vi "EVT HLP Set Frame Param.vi"(5 "convertBitDepth":i32, 6 "convertColor":i32, 7 "pixel_type":u32, 9 "size_y":u32, 10 "size_x":u32, 11 "frame":T1) -> (3 "frame out":T1)   [LabVIEW 2019, in "EmergentCameraC.lvlib"]
doc: "EMERGENTCAMERAC_API void EVT_HLP_SetFrameParam(EmergentFrame* frame, unsigned int size_x, unsigned int size_y, PIXEL_FORMAT pixel_type, int convertColor, int convertBitDepth);"
uses:
  EmergentCameraC.lvlib
  emergentInstall_Windows/win64/eSDK/bin/EmergentCameraC.dll
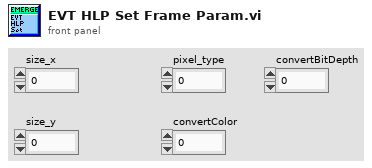
[diagram p1: front panel]
types:
  T1 = cluster{"pixel_type":u32, "size_x":u32, "size_y":u32, "stride":i32, "offset_x":u32, "offset_y":u32, "padding_x":u32, "padding_y":u32, "trailer_size_y":u32, "frame_id":u16, "@dummy control@":i8, "@dummy control@":i8, "imagePtr":i64, "bufferSize":u32, "@dummy control@":i8, "@dummy control@":i8, "@dummy control@":i8, "@dummy control@":i8, "timestamp":u64, "nsecs":u64, "convertColor":i32, "convertBitDepth":i32, "privateData[0]":u8, "privateData[1]":u8, "privateData[2]":u8, "privateData[3]":u8, "privateData[4]":u8, "privateData[5]":u8, "privateData[6]":u8, "privateData[7]":u8, "privateData[8]":u8, "privateData[9]":u8, "privateData[10]":u8, "privateData[11]":u8, "privateData[12]":u8, "privateData[13]":u8, "privateData[14]":u8, "privateData[15]":u8, "privateData[16]":u8, "privateData[17]":u8, "privateData[18]":u8, "privateData[19]":u8, "privateData[20]":u8, "privateData[21]":u8, "privateData[22]":u8, "privateData[23]":u8, "privateData[24]":u8, "privateData[25]":u8, "privateData[26]":u8, "privateData[27]":u8, "privateData[28]":u8, "privateData[29]":u8, "privateData[30]":u8, "privateData[31]":u8, "privateData[32]":u8, "privateData[33]":u8, "privateData[34]":u8, "privateData[35]":u8, "privateData[36]":u8, "privateData[37]":u8, "privateData[38]":u8, "privateData[39]":u8, "privateData[40]":u8, "privateData[41]":u8, "privateData[42]":u8, "privateData[43]":u8, "privateData[44]":u8, "privateData[45]":u8, "privateData[46]":u8, "privateData[47]":u8, "privateData[48]":u8, "privateData[49]":u8, "privateData[50]":u8, "privateData[51]":u8, "privateData[52]":u8, "privateData[53]":u8, "privateData[54]":u8, "privateData[55]":u8, "privateData[56]":u8, "privateData[57]":u8, "privateData[58]":u8, "privateData[59]":u8, "privateData[60]":u8, "privateData[61]":u8, "privateData[62]":u8, "privateData[63]":u8, "privateData[64]":u8, "privateData[65]":u8, "privateData[66]":u8, "privateData[67]":u8, "privateData[68]":u8, "privateData[69]":u8, "privateData[70]":u8, "privateData[71]":u8, "privateData[72]":u8, "privateData[73]":u8, "privateData[74]":u8, "privateData[75]":u8, "privateData[76]":u8, "privateData[77]":u8, "privateData[78]":u8, "privateData[79]":u8, "privateData[80]":u8, "privateData[81]":u8, "privateData[82]":u8, "privateData[83]":u8, "privateData[84]":u8, "privateData[85]":u8, "privateData[86]":u8, "privateData[87]":u8, "privateData[88]":u8, "privateData[89]":u8, "privateData[90]":u8, "privateData[91]":u8, "privateData[92]":u8, "privateData[93]":u8, "privateData[94]":u8, "privateData[95]":u8, "privateData[96]":u8, "privateData[97]":u8, "privateData[98]":u8, "privateData[99]":u8, "privateData[100]":u8, "privateData[101]":u8, "privateData[102]":u8, "privateData[103]":u8, "privateData[104]":u8, "privateData[105]":u8, "privateData[106]":u8, "privateData[107]":u8, "privateData[108]":u8, "privateData[109]":u8, "privateData[110]":u8, "privateData[111]":u8, "privateData[112]":u8, "privateData[113]":u8, "privateData[114]":u8, "privateData[115]":u8, "privateData[116]":u8, "privateData[117]":u8, "privateData[118]":u8, "privateData[119]":u8, "privateData[120]":u8, "privateData[121]":u8, "privateData[122]":u8, "privateData[123]":u8, "privateData[124]":u8, "privateData[125]":u8, "privateData[126]":u8, "privateData[127]":u8, "privateData[128]":u8, "privateData[129]":u8, "privateData[130]":u8, "privateData[131]":u8, "privateData[132]":u8, "privateData[133]":u8, "privateData[134]":u8, "privateData[135]":u8, "privateData[136]":u8, "privateData[137]":u8, "privateData[138]":u8, "privateData[139]":u8, "privateData[140]":u8, "privateData[141]":u8, "privateData[142]":u8, "privateData[143]":u8, "privateData[144]":u8, "privateData[145]":u8, "privateData[146]":u8, "privateData[147]":u8, "privateData[148]":u8, "privateData[149]":u8, "privateData[150]":u8, "privateData[151]":u8, "privateData[152]":u8, "privateData[153]":u8, "privateData[154]":u8, "privateData[155]":u8, "privateData[156]":u8, "privateData[157]":u8, "privateData[158]":u8, "privateData[159]":u8, "privateData[160]":u8, "privateData[161]":u8, "privateData[162]":u8, "privateData[163]":u8, "privateData[164]":u8, "privateData[165]":u8, "privateData[166]":u8, "privateData[167]":u8, "privateData[168]":u8, "privateData[169]":u8, "privateData[170]":u8, "privateData[171]":u8, "privateData[172]":u8, "privateData[173]":u8, "privateData[174]":u8, "privateData[175]":u8, "privateData[176]":u8, "privateData[177]":u8, "privateData[178]":u8, "privateData[179]":u8, "privateData[180]":u8, "privateData[181]":u8, "privateData[182]":u8, "privateData[183]":u8, "privateData[184]":u8, "privateData[185]":u8, "privateData[186]":u8, "privateData[187]":u8, "privateData[188]":u8, "privateData[189]":u8, "privateData[190]":u8, "privateData[191]":u8, "privateData[192]":u8, "privateData[193]":u8, "privateData[194]":u8, "privateData[195]":u8, "privateData[196]":u8, "privateData[197]":u8, "privateData[198]":u8, "privateData[199]":u8, "privateData[200]":u8, "privateData[201]":u8, "privateData[202]":u8, "privateData[203]":u8, "privateData[204]":u8, "privateData[205]":u8, "privateData[206]":u8, "privateData[207]":u8, "privateData[208]":u8, "privateData[209]":u8, "privateData[210]":u8, "privateData[211]":u8, "privateData[212]":u8, "privateData[213]":u8, "privateData[214]":u8, "privateData[215]":u8, "privateData[216]":u8, "privateData[217]":u8, "privateData[218]":u8, "privateData[219]":u8, "privateData[220]":u8, "privateData[221]":u8, "privateData[222]":u8, "privateData[223]":u8, "privateData[224]":u8, "privateData[225]":u8, "privateData[226]":u8, "privateData[227]":u8, "privateData[228]":u8, "privateData[229]":u8, "privateData[230]":u8, "privateData[231]":u8, "privateData[232]":u8, "privateData[233]":u8, "privateData[234]":u8, "privateData[235]":u8, "privateData[236]":u8, "privateData[237]":u8, "privateData[238]":u8, "privateData[239]":u8, "privateData[240]":u8, "privateData[241]":u8, "privateData[242]":u8, "privateData[243]":u8, "privateData[244]":u8, "privateData[245]":u8, "privateData[246]":u8, "privateData[247]":u8, "privateData[248]":u8, "privateData[249]":u8, "privateData[250]":u8, "privateData[251]":u8, "privateData[252]":u8, "privateData[253]":u8, "privateData[254]":u8, "privateData[255]":u8}
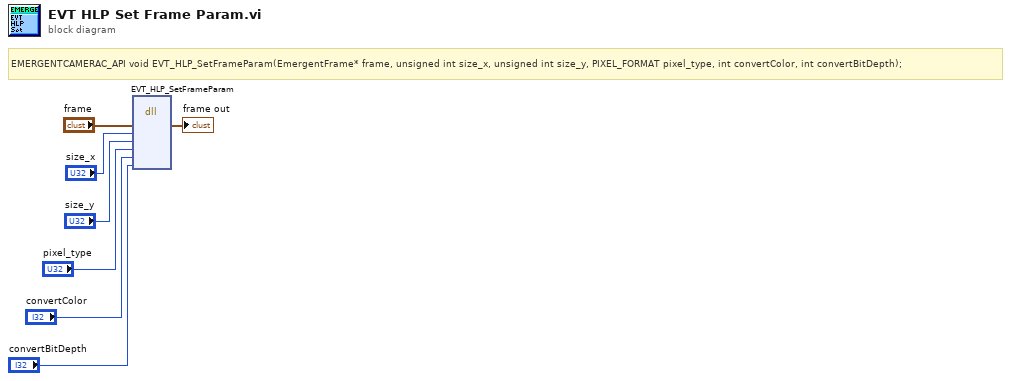
[diagram p0: block diagram]
diagram:
  # "EMERGENTCAMERAC_API void EVT_HLP_SetFrameParam(EmergentFrame* frame, unsigned int size_x, unsigned int size_y, PIXEL_FORMAT pixel_type, int convertColor, int convertBitDepth);"
  n1 = dll-call lib="E:/emergent/host-new_QT/emergentInstall_Windows/win64/eSDK/bin/EmergentCameraC.*" fn="EVT_HLP_SetFrameParam"("frame"="frame", "size_x"="size_x", "size_y"="size_y", "pixel_type"="pixel_type", "convertColor"="convertColor", "convertBitDepth"="convertBitDepth") -> ("frame"=→"frame out":T1)  [unwired: 9 in, 2 out]
